vi "GetAlarms.vi"(0 "Device in":refnum<class "Device.lvclass">, 11 "error in (no error)":errorcluster) -> (4 "Device out":refnum<class "Device.lvclass">, 6 "Alarm":bool, 8 "Warning":bool, 15 "error out":errorcluster)   [LabVIEW 2019, in "Device.lvclass"]
uses:
  Device.lvclass
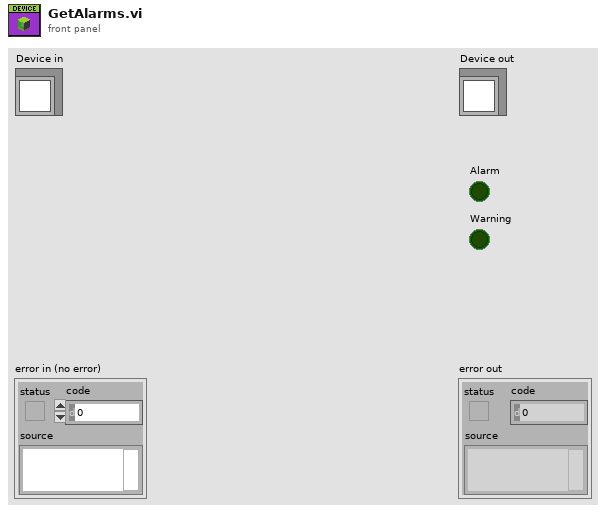
[diagram p1: front panel]
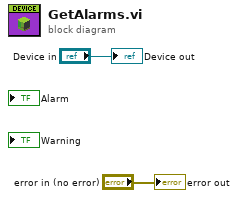
[diagram p0: block diagram]
diagram:
  "error out" <- "error in (no error)"
  "Device out" <- "Device in"
